vi "setOpenBottom.vi"(0 "reference":refnum<class "CallNode.lvclass">, 1 "openBottom":bool, 5 "error in (no error)":errorcluster) -> (14 "reference out":refnum<class "CallNode.lvclass">, 19 "error out":errorcluster)   [LabVIEW 2012, in "CallNode.lvclass"]
doc: "public void setOpenBottom(boolean newValue)"
uses:
  <resource>/Framework/Providers/Open_GDS/UML/CallNode_class/CallNode.lvclass
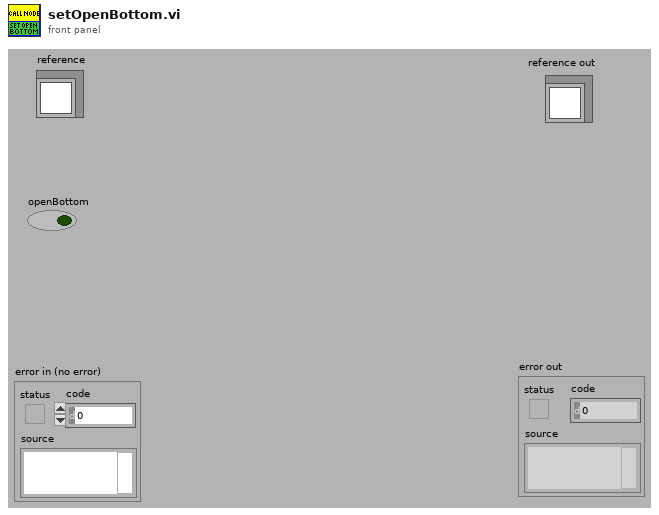
[diagram p1: front panel]
types:
  T1 = typedef "CallNode.lvclass/ObjectAttributes.ctl" = cluster{"Base class":T2, "objectCallNodeRef":refnum<class "AbstractNode.lvclass">, "signaled":bool, "openBottom":bool, "DEFAULT_WIDTH":i32, "DEFAULT_HEIGHT":i32, "CALL_YGAP":i32}
  T2 = typedef "RectangularNode.lvclass/ObjectAttributes.ctl" = cluster{"Base class":T3, "bounds":T4}
  T3 = typedef "AbstractNode.lvclass/ObjectAttributes.ctl" = cluster{"parent":refnum<class "AbstractNode.lvclass">, "children":refnum<class "AbstractNode.lvclass">[], "Hidden":bool}
  T4 = typedef "Rectangle Rectangle2D.ctl" = cluster{"x":dbl, "y":dbl, "width":dbl, "height":dbl}
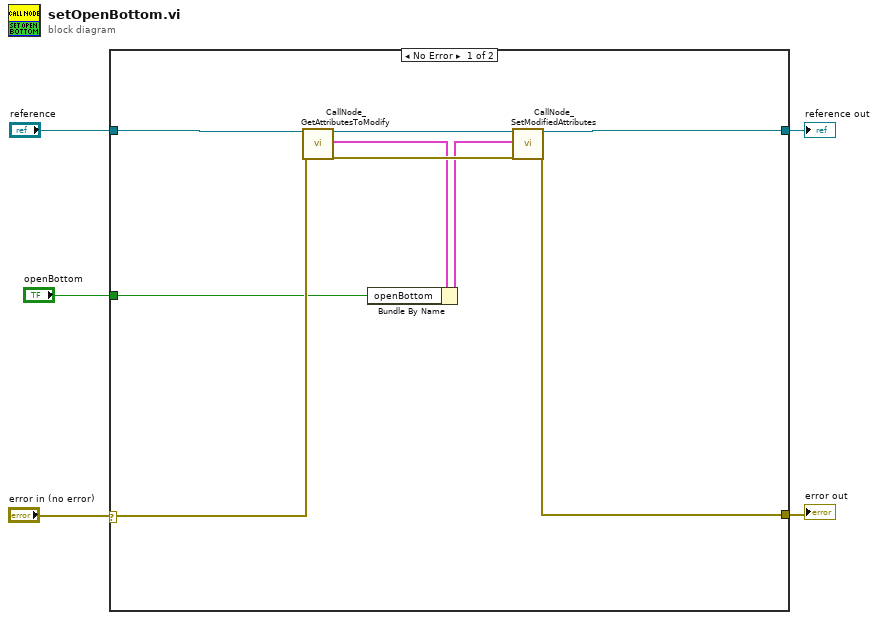
[diagram p0: block diagram]
diagram:
  n1 = case shown="No Error" "error in (no error)" {
    selector: "error in (no error)" -> [w11 w15]
    tunnel: "reference" -> [w14 w16]
    tunnel: [w13 w15] -> w4
    tunnel: [w12 w16] -> w3
    tunnel: "openBottom" -> [w10 _]
    frame No Error {
      n2 = call <resource>:"CallNode_GetAttributesToModify.vi"("reference in"=w14, "error in (no error)"=w11) -> ("reference out"=w9:refnum<class "CallNode.lvclass">, "Attributes"=w6:T1, "error out"=w8:errorcluster)  [unwired: 1 in, 14 out]
      n3 = Bundle By Name(cluster=w6, "openBottom"=w10) -> (w7:T1)
      n4 = call <resource>:"CallNode_SetModifiedAttributes.vi"("reference in"=w9, "Attributes"=w7, "error in (no error)"=w8) -> ("reference out"=w12:refnum<class "CallNode.lvclass">, "error out"=w13:errorcluster)  [unwired: 3 in, 12 out]
    }
    frame Error {
    }
  }
  "reference out" <- w3
  "error out" <- w4
